vi "check operator action.vi"(9 "Motion Steps in":string[](array[string]), 10 "Part Type":string, 11 "input cluster":T3={"AT glass position"={"Tag Name"="S060.PXI.Signals.PlltData.SN", "Network Path"="172.15.51.1,1,0", "use opc"=FALSE, "DataSocket Reference"={"CWDSLib._DCWDataSocket"=refnum, "CWDSLib._DCWData"=refnum, "OnDataUpdated"=0, "OnStatusUpdated"=0}}, "AT shade position"={"Tag Name"="S060.PXI.Signals.PlltData.SN", "Network Path"="172.15.51.1,1,0", "use opc"=FALSE, "DataSocket Reference"={"CWDSLib._DCWDataSocket"=refnum, "CWDSLib._DCWData"=refnum, "OnDataUpdated"=0, "OnStatusUpdated"=0}}, "AT in glass wand lower pos"={"Tag Name"="S060.PXI.Signals.PlltData.SN", "Network Path"="172.15.51.1,1,0", "use opc"=FALSE, "DataSocket Reference"={"CWDSLib._DCWDataSocket"=refnum, "CWDSLib._DCWData"=refnum, "OnDataUpdated"=0, "OnStatusUpdated"=0}}, "AT in glass wand up pos"={"Tag Name"="S060.PXI.Signals.PlltData.SN", "Network Path"="172.15.51.1,1,0", "use opc"=FALSE, "DataSocket Reference"={"CWDSLib._DCWDataSocket"=refnum, "CWDSLib._DCWData"=refnum, "OnDataUpdated"=0, "OnStatusUpdated"=0}}, "AT in sunshad wand lower pos"={"Tag Name"="S060.PXI.Signals.PlltData.SN", "Network Path"="172.15.51.1,1,0", "use opc"=FALSE, "DataSocket Reference"={"CWDSLib._DCWDataSocket"=refnum, "CWDSLib._DCWData"=refnum, "OnDataUpdated"=0, "OnStatusUpdated"=0}}, "AT in sunshad wand up pos"={"Tag Name"="S060.PXI.Signals.PlltData.SN", "Network Path"="172.15.51.1,1,0", "use opc"=FALSE, "DataSocket Reference"={"CWDSLib._DCWDataSocket"=refnum, "CWDSLib._DCWData"=refnum, "OnDataUpdated"=0, "OnStatusUpdated"=0}}, "AT in wand home pos"={"Tag Name"="S060.PXI.Signals.PlltData.SN", "Network Path"="172.15.51.1,1,0", "use opc"=FALSE, "DataSocket Reference"={"CWDSLib._DCWDataSocket"=refnum, "CWDSLib._DCWData"=refnum, "OnDataUpdated"=0, "OnStatusUpdated"=0}}, "LVDT's Extended"={"Tag Name"="S060.PXI.Signals.PlltData.SN", "Network Path"="172.15.51.1,1,0", "use opc"=FALSE, "DataSocket Reference"={"CWDSLib._DCWDataSocket"=refnum, "CWDSLib._DCWData"=refnum, "OnDataUpdated"=0, "OnStatusUpdated"=0}}, "bolt check 1"={"Tag Name"="S060.PXI.Signals.PlltData.SN", "Network Path"="172.15.51.1,1,0", "use opc"=FALSE, "DataSocket Reference"={"CWDSLib._DCWDataSocket"=refnum, "CWDSLib._DCWData"=refnum, "OnDataUpdated"=0, "OnStatusUpdated"=0}}, "bolt check 2"={"Tag Name"="S060.PXI.Signals.PlltData.SN", "Network Path"="172.15.51.1,1,0", "use opc"=FALSE, "DataSocket Reference"={"CWDSLib._DCWDataSocket"=refnum, "CWDSLib._DCWData"=refnum, "OnDataUpdated"=0, "OnStatusUpdated"=0}}, "bolt check 3"={"Tag Name"="S060.PXI.Signals.PlltData.SN", "Network Path"="172.15.51.1,1,0", "use opc"=FALSE, "DataSocket Reference"={"CWDSLib._DCWDataSocket"=refnum, "CWDSLib._DCWData"=refnum, "OnDataUpdated"=0, "OnStatusUpdated"=0}}, "bolt check 4"={"Tag Name"="S060.PXI.Signals.PlltData.SN", "Network Path"="172.15.51.1,1,0", "use opc"=FALSE, "DataSocket Reference"={"CWDSLib._DCWDataSocket"=refnum, "CWDSLib._DCWData"=refnum, "OnDataUpdated"=0, "OnStatusUpdated"=0}}, "bolt check 5"={"Tag Name"="S060.PXI.Signals.PlltData.SN", "Network Path"="172.15.51.1,1,0", "use opc"=FALSE, "DataSocket Reference"={"CWDSLib._DCWDataSocket"=refnum, "CWDSLib._DCWData"=refnum, "OnDataUpdated"=0, "OnStatusUpdated"=0}}, "bolt check 6"={"Tag Name"="S060.PXI.Signals.PlltData.SN", "Network Path"="172.15.51.1,1,0", "use opc"=FALSE, "DataSocket Reference"={"CWDSLib._DCWDataSocket"=refnum, "CWDSLib._DCWData"=refnum, "OnDataUpdated"=0, "OnStatusUpdated"=0}}, "bolt check 7"={"Tag Name"="S060.PXI.Signals.PlltData.SN", "Network Path"="172.15.51.1,1,0", "use opc"=FALSE, "DataSocket Reference"={"CWDSLib._DCWDataSocket"=refnum, "CWDSLib._DCWData"=refnum, "OnDataUpdated"=0, "OnStatusUpdated"=0}}, "bolt check 8"={"Tag Name"="S060.PXI.Signals.PlltData.SN", "Network Path"="172.15.51.1,1,0", "use opc"=FALSE, "DataSocket Reference"={"CWDSLib._DCWDataSocket"=refnum, "CWDSLib._DCWData"=refnum, "OnDataUpdated"=0, "OnStatusUpdated"=0}}, "start"={"Tag Name"="S060.PXI.Signals.PlltData.SN", "Network Path"="172.15.51.1,1,0", "use opc"=FALSE, "DataSocket Reference"={"CWDSLib._DCWDataSocket"=refnum, "CWDSLib._DCWData"=refnum, "OnDataUpdated"=0, "OnStatusUpdated"=0}}, "abort"={"Tag Name"="S060.PXI.Signals.PlltData.SN", "Network Path"="172.15.51.1,1,0", "use opc"=FALSE, "DataSocket Reference"={"CWDSLib._DCWDataSocket"=refnum, "CWDSLib._DCWData"=refnum, "OnDataUpdated"=0, "OnStatusUpdated"=0}}, "LVDT's Retracted"={"Tag Name"="S060.PXI.Signals.PlltData.SN", "Network Path"="172.15.51.1,1,0", "use opc"=FALSE, "DataSocket Reference"={"CWDSLib._DCWDataSocket"=refnum, "CWDSLib._DCWData"=refnum, "OnDataUpdated"=0, "OnStatusUpdated"=0}}, "manual barcode print"={"Tag Name"="S060.PXI.Signals.PlltData.SN", "Network Path"="172.15.51.1,1,0", "use opc"=FALSE, "DataSocket Reference"={"CWDSLib._DCWDataSocket"=refnum, "CWDSLib._DCWData"=refnum, "OnDataUpdated"=0, "OnStatusUpdated"=0}}, "ss servo at open"={"Tag Name"="S060.PXI.Signals.PlltData.SN", "Network Path"="172.15.51.1,1,0", "use opc"=FALSE, "DataSocket Reference"={"CWDSLib._DCWDataSocket"=refnum, "CWDSLib._DCWData"=refnum, "OnDataUpdated"=0, "OnStatusUpdated"=0}}, "ss servo at close"={"Tag Name"="S060.PXI.Signals.PlltData.SN", "Network Path"="172.15.51.1,1,0", "use opc"=FALSE, "DataSocket Reference"={"CWDSLib._DCWDataSocket"=refnum, "CWDSLib._DCWData"=refnum, "OnDataUpdated"=0, "OnStatusUpdated"=0}}, "ss servo opening"={"Tag Name"="S060.PXI.Signals.PlltData.SN", "Network Path"="172.15.51.1,1,0", "use opc"=FALSE, "DataSocket Reference"={"CWDSLib._DCWDataSocket"=refnum, "CWDSLib._DCWData"=refnum, "OnDataUpdated"=0, "OnStatusUpdated"=0}}, "ss servo closing"={"Tag Name"="S060.PXI.Signals.PlltData.SN", "Network Path"="172.15.51.1,1,0", "use opc"=FALSE, "DataSocket Reference"={"CWDSLib._DCWDataSocket"=refnum, "CWDSLib._DCWData"=refnum, "OnDataUpdated"=0, "OnStatusUpdated"=0}}, "control slide at home"={"Tag Name"="S060.PXI.Signals.PlltData.SN", "Network Path"="172.15.51.1,1,0", "use opc"=FALSE, "DataSocket Reference"={"CWDSLib._DCWDataSocket"=refnum, "CWDSLib._DCWData"=refnum, "OnDataUpdated"=0, "OnStatusUpdated"=0}}, "control slide left good"={"Tag Name"="S060.PXI.Signals.PlltData.SN", "Network Path"="172.15.51.1,1,0", "use opc"=FALSE, "DataSocket Reference"={"CWDSLib._DCWDataSocket"=refnum, "CWDSLib._DCWData"=refnum, "OnDataUpdated"=0, "OnStatusUpdated"=0}}, "control slide left over stroke"={"Tag Name"="S060.PXI.Signals.PlltData.SN", "Network Path"="172.15.51.1,1,0", "use opc"=FALSE, "DataSocket Reference"={"CWDSLib._DCWDataSocket"=refnum, "CWDSLib._DCWData"=refnum, "OnDataUpdated"=0, "OnStatusUpdated"=0}}, "control slide right good"={"Tag Name"="S060.PXI.Signals.PlltData.SN", "Network Path"="172.15.51.1,1,0", "use opc"=FALSE, "DataSocket Reference"={"CWDSLib._DCWDataSocket"=refnum, "CWDSLib._DCWData"=refnum, "OnDataUpdated"=0, "OnStatusUpdated"=0}}, "control slide right over stroke"={"Tag Name"="S060.PXI.Signals.PlltData.SN", "Network Path"="172.15.51.1,1,0", "use opc"=FALSE, "DataSocket Reference"={"CWDSLib._DCWDataSocket"=refnum, "CWDSLib._DCWData"=refnum, "OnDataUpdated"=0, "OnStatusUpdated"=0}}, "wind deflector high speed pos"={"Tag Name"="S060.PXI.Signals.PlltData.SN", "Network Path"="172.15.51.1,1,0", "use opc"=FALSE, "DataSocket Reference"={"CWDSLib._DCWDataSocket"=refnum, "CWDSLib._DCWData"=refnum, "OnDataUpdated"=0, "OnStatusUpdated"=0}}, "wind deflector low speed pos"={"Tag Name"="S060.PXI.Signals.PlltData.SN", "Network Path"="172.15.51.1,1,0", "use opc"=FALSE, "DataSocket Reference"={"CWDSLib._DCWDataSocket"=refnum, "CWDSLib._DCWData"=refnum, "OnDataUpdated"=0, "OnStatusUpdated"=0}}, "AT VentPMACatHome"={"Tag Name"="S060.PXI.Signals.PlltData.SN", "Network Path"="172.15.51.1,1,0", "use opc"=FALSE, "DataSocket Reference"={"CWDSLib._DCWDataSocket"=refnum, "CWDSLib._DCWData"=refnum, "OnDataUpdated"=0, "OnStatusUpdated"=0}}, "AT VentPMACisExtend"={"Tag Name"="S060.PXI.Signals.PlltData.SN", "Network Path"="172.15.51.1,1,0", "use opc"=FALSE, "DataSocket Reference"={"CWDSLib._DCWDataSocket"=refnum, "CWDSLib._DCWData"=refnum, "OnDataUpdated"=0, "OnStatusUpdated"=0}}, "SS Barcode Scanner Bypassed"={"Tag Name"="S060.PXI.Signals.PlltData.SN", "Network Path"="172.15.51.1,1,0", "use opc"=FALSE, "DataSocket Reference"={"CWDSLib._DCWDataSocket"=refnum, "CWDSLib._DCWData"=refnum, "OnDataUpdated"=0, "OnStatusUpdated"=0}}, "Check Frame Barcode"={"Tag Name"="S060.PXI.Signals.PlltData.SN", "Network Path"="172.15.51.1,1,0", "use opc"=FALSE, "DataSocket Reference"={"CWDSLib._DCWDataSocket"=refnum, "CWDSLib._DCWData"=refnum, "OnDataUpdated"=0, "OnStatusUpdated"=0}}, "Z LVDTs Extended"={"Tag Name"="S060.PXI.Signals.PlltData.SN", "Network Path"="172.15.51.1,1,0", "use opc"=FALSE, "DataSocket Reference"={"CWDSLib._DCWDataSocket"=refnum, "CWDSLib._DCWData"=refnum, "OnDataUpdated"=0, "OnStatusUpdated"=0}}, "NVH Operator Pass"={"Tag Name"="S060.PXI.Signals.PlltData.SN", "Network Path"="172.15.51.1,1,0", "use opc"=FALSE, "DataSocket Reference"={"CWDSLib._DCWDataSocket"=refnum, "CWDSLib._DCWData"=refnum, "OnDataUpdated"=0, "OnStatusUpdated"=0}}, "NVH Operator Fail"={"Tag Name"="S060.PXI.Signals.PlltData.SN", "Network Path"="172.15.51.1,1,0", "use opc"=FALSE, "DataSocket Reference"={"CWDSLib._DCWDataSocket"=refnum, "CWDSLib._DCWData"=refnum, "OnDataUpdated"=0, "OnStatusUpdated"=0}}, "NVH Operator Express Glass Open"={"Tag Name"="S060.PXI.Signals.PlltData.SN", "Network Path"="172.15.51.1,1,0", "use opc"=FALSE, "DataSocket Reference"={"CWDSLib._DCWDataSocket"=refnum, "CWDSLib._DCWData"=refnum, "OnDataUpdated"=0, "OnStatusUpdated"=0}}, "NVH Operator Express Glass Close"={"Tag Name"="S060.PXI.Signals.PlltData.SN", "Network Path"="172.15.51.1,1,0", "use opc"=FALSE, "DataSocket Reference"={"CWDSLib._DCWDataSocket"=refnum, "CWDSLib._DCWData"=refnum, "OnDataUpdated"=0, "OnStatusUpdated"=0}}, "NVH Operator Express Rollo Open01"={"Tag Name"="S060.PXI.Signals.PlltData.SN", "Network Path"="172.15.51.1,1,0", "use opc"=FALSE, "DataSocket Reference"={"CWDSLib._DCWDataSocket"=refnum, "CWDSLib._DCWData"=refnum, "OnDataUpdated"=0, "OnStatusUpdated"=0}}, "NVH Operator Express Rollo Close01"={"Tag Name"="S060.PXI.Signals.PlltData.SN", "Network Path"="172.15.51.1,1,0", "use opc"=FALSE, "DataSocket Reference"={"CWDSLib._DCWDataSocket"=refnum, "CWDSLib._DCWData"=refnum, "OnDataUpdated"=0, "OnStatusUpdated"=0}}, "NVH Operator Express Rollo Open02"={"Tag Name"="S060.PXI.Signals.PlltData.SN", "Network Path"="172.15.51.1,1,0", "use opc"=FALSE, "DataSocket Reference"={"CWDSLib._DCWDataSocket"=refnum, "CWDSLib._DCWData"=refnum, "OnDataUpdated"=0, "OnStatusUpdated"=0}}, "NVH Operator Express Rollo Close02"={"Tag Name"="S060.PXI.Signals.PlltData.SN", "Network Path"="172.15.51.1,1,0", "use opc"=FALSE, "DataSocket Reference"={"CWDSLib._DCWDataSocket"=refnum, "CWDSLib._DCWData"=refnum, "OnDataUpdated"=0, "OnStatusUpdated"=0}}, "NVH Operator Vent Open Noise"={"Tag Name"="S060.PXI.Signals.PlltData.SN", "Network Path"="172.15.51.1,1,0", "use opc"=FALSE, "DataSocket Reference"={"CWDSLib._DCWDataSocket"=refnum, "CWDSLib._DCWData"=refnum, "OnDataUpdated"=0, "OnStatusUpdated"=0}}, "NVH Operator Vent Close Noise"={"Tag Name"="S060.PXI.Signals.PlltData.SN", "Network Path"="172.15.51.1,1,0", "use opc"=FALSE, "DataSocket Reference"={"CWDSLib._DCWDataSocket"=refnum, "CWDSLib._DCWData"=refnum, "OnDataUpdated"=0, "OnStatusUpdated"=0}}, "NVH Operator Sunshade Open Noise"={"Tag Name"="S060.PXI.Signals.PlltData.SN", "Network Path"="172.15.51.1,1,0", "use opc"=FALSE, "DataSocket Reference"={"CWDSLib._DCWDataSocket"=refnum, "CWDSLib._DCWData"=refnum, "OnDataUpdated"=0, "OnStatusUpdated"=0}}, "NVH Operator Sunshade Close Noise"={"Tag Name"="S060.PXI.Signals.PlltData.SN", "Network Path"="172.15.51.1,1,0", "use opc"=FALSE, "DataSocket Reference"={"CWDSLib._DCWDataSocket"=refnum, "CWDSLib._DCWData"=refnum, "OnDataUpdated"=0, "OnStatusUpdated"=0}}, "NVH Operator Glass Open Noise"={"Tag Name"="S060.PXI.Signals.PlltData.SN", "Network Path"="172.15.51.1,1,0", "use opc"=FALSE, "DataSocket Reference"={"CWDSLib._DCWDataSocket"=refnum, "CWDSLib._DCWData"=refnum, "OnDataUpdated"=0, "OnStatusUpdated"=0}}, "NVH Operator Glass Close Noise"={"Tag Name"="S060.PXI.Signals.PlltData.SN", "Network Path"="172.15.51.1,1,0", "use opc"=FALSE, "DataSocket Reference"={"CWDSLib._DCWDataSocket"=refnum, "CWDSLib._DCWData"=refnum, "OnDataUpdated"=0, "OnStatusUpdated"=0}}, "NVH Operator Finish"={"Tag Name"="S060.PXI.Signals.PlltData.SN", "Network Path"="172.15.51.1,1,0", "use opc"=FALSE, "DataSocket Reference"={"CWDSLib._DCWDataSocket"=refnum, "CWDSLib._DCWData"=refnum, "OnDataUpdated"=0, "OnStatusUpdated"=0}}, "NVH Operator Check"={"Tag Name"="S060.PXI.Signals.PlltData.SN", "Network Path"="172.15.51.1,1,0", "use opc"=FALSE, "DataSocket Reference"={"CWDSLib._DCWDataSocket"=refnum, "CWDSLib._DCWData"=refnum, "OnDataUpdated"=0, "OnStatusUpdated"=0}}, "windproof position"={"Tag Name"="S060.PXI.Signals.PlltData.SN", "Network Path"="172.15.51.1,1,0", "use opc"=FALSE, "DataSocket Reference"={"CWDSLib._DCWDataSocket"=refnum, "CWDSLib._DCWData"=refnum, "OnDataUpdated"=0, "OnStatusUpdated"=0}}, "NVH Operator Express Glass vent Open"={"Tag Name"="S060.PXI.Signals.PlltData.SN", "Network Path"="172.15.51.1,1,0", "use opc"=FALSE, "DataSocket Reference"={"CWDSLib._DCWDataSocket"=refnum, "CWDSLib._DCWData"=refnum, "OnDataUpdated"=0, "OnStatusUpdated"=0}}, "NVH Operator Express Glass Vent Close"={"Tag Name"="S060.PXI.Signals.PlltData.SN", "Network Path"="172.15.51.1,1,0", "use opc"=FALSE, "DataSocket Reference"={"CWDSLib._DCWDataSocket"=refnum, "CWDSLib._DCWData"=refnum, "OnDataUpdated"=0, "OnStatusUpdated"=0}}, "NVH Operator Re-do"={"Tag Name"="S060.PXI.Signals.PlltData.SN", "Network Path"="172.15.51.1,1,0", "use opc"=FALSE, "DataSocket Reference"={"CWDSLib._DCWDataSocket"=refnum, "CWDSLib._DCWData"=refnum, "OnDataUpdated"=0, "OnStatusUpdated"=0}}, "AT at vent ATS test pos"={"Tag Name"="S060.PXI.Signals.PlltData.SN", "Network Path"="172.15.51.1,1,0", "use opc"=FALSE, "DataSocket Reference"={"CWDSLib._DCWDataSocket"=refnum, "CWDSLib._DCWData"=refnum, "OnDataUpdated"=0, "OnStatusUpdated"=0}}, "AT at vent ATS Home pos"={"Tag Name"="S060.PXI.Signals.PlltData.SN", "Network Path"="172.15.51.1,1,0", "use opc"=FALSE, "DataSocket Reference"={"CWDSLib._DCWDataSocket"=refnum, "CWDSLib._DCWData"=refnum, "OnDataUpdated"=0, "OnStatusUpdated"=0}}, "Start Adjust LVDT"={"Tag Name"="S060.PXI.Signals.PlltData.SN", "Network Path"="172.15.51.1,1,0", "use opc"=FALSE, "DataSocket Reference"={"CWDSLib._DCWDataSocket"=refnum, "CWDSLib._DCWData"=refnum, "OnDataUpdated"=0, "OnStatusUpdated"=0}}, "Finish Adjust LVDT"={"Tag Name"="S060.PXI.Signals.PlltData.SN", "Network Path"="172.15.51.1,1,0", "use opc"=FALSE, "DataSocket Reference"={"CWDSLib._DCWDataSocket"=refnum, "CWDSLib._DCWData"=refnum, "OnDataUpdated"=0, "OnStatusUpdated"=0}}} {"AT in sunshad wand up pos"."DataSocket Reference"."OnStatusUpdated" format="%.0x"; "AT in sunshad wand up pos"."DataSocket Reference"."OnDataUpdated" format="%.0x"; "AT in glass wand up pos"."DataSocket Reference"."OnStatusUpdated" format="%.0x"; "AT in glass wand up pos"."DataSocket Reference"."OnDataUpdated" format="%.0x"; "Finish Adjust LVDT"."DataSocket Reference"."OnStatusUpdated" format="%.0x"; "Finish Adjust LVDT"."DataSocket Reference"."OnDataUpdated" format="%.0x"; "Start Adjust LVDT"."DataSocket Reference"."OnStatusUpdated" format="%.0x"; "Start Adjust LVDT"."DataSocket Reference"."OnDataUpdated" format="%.0x"; "AT at vent ATS Home pos"."DataSocket Reference"."OnStatusUpdated" format="%.0x"; "AT at vent ATS Home pos"."DataSocket Reference"."OnDataUpdated" format="%.0x"; "AT at vent ATS test pos"."DataSocket Reference"."OnStatusUpdated" format="%.0x"; "AT at vent ATS test pos"."DataSocket Reference"."OnDataUpdated" format="%.0x"; "NVH Operator Re-do"."DataSocket Reference"."OnStatusUpdated" format="%.0x"; "NVH Operator Re-do"."DataSocket Reference"."OnDataUpdated" format="%.0x"; "NVH Operator Express Glass Vent Close"."DataSocket Reference"."OnStatusUpdated" format="%.0x"; "NVH Operator Express Glass Vent Close"."DataSocket Reference"."OnDataUpdated" format="%.0x"; "NVH Operator Express Glass vent Open"."DataSocket Reference"."OnStatusUpdated" format="%.0x"; "NVH Operator Express Glass vent Open"."DataSocket Reference"."OnDataUpdated" format="%.0x"; "windproof position"."DataSocket Reference"."OnStatusUpdated" format="%.0x"; "windproof position"."DataSocket Reference"."OnDataUpdated" format="%.0x"; "NVH Operator Check"."DataSocket Reference"."OnStatusUpdated" format="%.0x"; "NVH Operator Check"."DataSocket Reference"."OnDataUpdated" format="%.0x"; "NVH Operator Finish"."DataSocket Reference"."OnStatusUpdated" format="%.0x"; "NVH Operator Finish"."DataSocket Reference"."OnDataUpdated" format="%.0x"; "NVH Operator Glass Close Noise"."DataSocket Reference"."OnStatusUpdated" format="%.0x"; "NVH Operator Glass Close Noise"."DataSocket Reference"."OnDataUpdated" format="%.0x"; "NVH Operator Glass Open Noise"."DataSocket Reference"."OnStatusUpdated" format="%.0x"; "NVH Operator Glass Open Noise"."DataSocket Reference"."OnDataUpdated" format="%.0x"; "NVH Operator Sunshade Close Noise"."DataSocket Reference"."OnStatusUpdated" format="%.0x"; "NVH Operator Sunshade Close Noise"."DataSocket Reference"."OnDataUpdated" format="%.0x"; "NVH Operator Sunshade Open Noise"."DataSocket Reference"."OnStatusUpdated" format="%.0x"; "NVH Operator Sunshade Open Noise"."DataSocket Reference"."OnDataUpdated" format="%.0x"; "NVH Operator Vent Close Noise"."DataSocket Reference"."OnStatusUpdated" format="%.0x"; "NVH Operator Vent Close Noise"."DataSocket Reference"."OnDataUpdated" format="%.0x"; "NVH Operator Vent Open Noise"."DataSocket Reference"."OnStatusUpdated" format="%.0x"; "NVH Operator Vent Open Noise"."DataSocket Reference"."OnDataUpdated" format="%.0x"; "NVH Operator Express Rollo Close02"."DataSocket Reference"."OnStatusUpdated" format="%.0x"; "NVH Operator Express Rollo Close02"."DataSocket Reference"."OnDataUpdated" format="%.0x"; "NVH Operator Express Rollo Open02"."DataSocket Reference"."OnStatusUpdated" format="%.0x"; "NVH Operator Express Rollo Open02"."DataSocket Reference"."OnDataUpdated" format="%.0x"; "NVH Operator Express Rollo Close01"."DataSocket Reference"."OnStatusUpdated" format="%.0x"; "NVH Operator Express Rollo Close01"."DataSocket Reference"."OnDataUpdated" format="%.0x"; "NVH Operator Express Rollo Open01"."DataSocket Reference"."OnStatusUpdated" format="%.0x"; "NVH Operator Express Rollo Open01"."DataSocket Reference"."OnDataUpdated" format="%.0x"; "NVH Operator Express Glass Close"."DataSocket Reference"."OnStatusUpdated" format="%.0x"; "NVH Operator Express Glass Close"."DataSocket Reference"."OnDataUpdated" format="%.0x"; "NVH Operator Express Glass Open"."DataSocket Reference"."OnStatusUpdated" format="%.0x"; "NVH Operator Express Glass Open"."DataSocket Reference"."OnDataUpdated" format="%.0x"; "NVH Operator Fail"."DataSocket Reference"."OnStatusUpdated" format="%.0x"; "NVH Operator Fail"."DataSocket Reference"."OnDataUpdated" format="%.0x"; "NVH Operator Pass"."DataSocket Reference"."OnStatusUpdated" format="%.0x"; "NVH Operator Pass"."DataSocket Reference"."OnDataUpdated" format="%.0x"; "Z LVDTs Extended"."DataSocket Reference"."OnStatusUpdated" format="%.0x"; "Z LVDTs Extended"."DataSocket Reference"."OnDataUpdated" format="%.0x"; "Check Frame Barcode"."DataSocket Reference"."OnStatusUpdated" format="%.0x"; "Check Frame Barcode"."DataSocket Reference"."OnDataUpdated" format="%.0x"; "SS Barcode Scanner Bypassed"."DataSocket Reference"."OnStatusUpdated" format="%.0x"; "SS Barcode Scanner Bypassed"."DataSocket Reference"."OnDataUpdated" format="%.0x"; "AT VentPMACisExtend"."DataSocket Reference"."OnStatusUpdated" format="%.0x"; "AT VentPMACisExtend"."DataSocket Reference"."OnDataUpdated" format="%.0x"; "AT VentPMACatHome"."DataSocket Reference"."OnStatusUpdated" format="%.0x"; "AT VentPMACatHome"."DataSocket Reference"."OnDataUpdated" format="%.0x"; "wind deflector low speed pos"."DataSocket Reference"."OnStatusUpdated" format="%.0x"; "wind deflector low speed pos"."DataSocket Reference"."OnDataUpdated" format="%.0x"; "wind deflector high speed pos"."DataSocket Reference"."OnStatusUpdated" format="%.0x"; "wind deflector high speed pos"."DataSocket Reference"."OnDataUpdated" format="%.0x"; "control slide right over stroke"."DataSocket Reference"."OnStatusUpdated" format="%.0x"; "control slide right over stroke"."DataSocket Reference"."OnDataUpdated" format="%.0x"; "control slide right good"."DataSocket Reference"."OnStatusUpdated" format="%.0x"; "control slide right good"."DataSocket Reference"."OnDataUpdated" format="%.0x"; "control slide left over stroke"."DataSocket Reference"."OnStatusUpdated" format="%.0x"; "control slide left over stroke"."DataSocket Reference"."OnDataUpdated" format="%.0x"; "control slide left good"."DataSocket Reference"."OnStatusUpdated" format="%.0x"; "control slide left good"."DataSocket Reference"."OnDataUpdated" format="%.0x"; "control slide at home"."DataSocket Reference"."OnStatusUpdated" format="%.0x"; "control slide at home"."DataSocket Reference"."OnDataUpdated" format="%.0x"; "ss servo closing"."DataSocket Reference"."OnStatusUpdated" format="%.0x"; "ss servo closing"."DataSocket Reference"."OnDataUpdated" format="%.0x"; "ss servo opening"."DataSocket Reference"."OnStatusUpdated" format="%.0x"; "ss servo opening"."DataSocket Reference"."OnDataUpdated" format="%.0x"; "ss servo at close"."DataSocket Reference"."OnStatusUpdated" format="%.0x"; "ss servo at close"."DataSocket Reference"."OnDataUpdated" format="%.0x"; "ss servo at open"."DataSocket Reference"."OnStatusUpdated" format="%.0x"; "ss servo at open"."DataSocket Reference"."OnDataUpdated" format="%.0x"; "manual barcode print"."DataSocket Reference"."OnStatusUpdated" format="%.0x"; "manual barcode print"."DataSocket Reference"."OnDataUpdated" format="%.0x"; "LVDT's Retracted"."DataSocket Reference"."OnStatusUpdated" format="%.0x"; "LVDT's Retracted"."DataSocket Reference"."OnDataUpdated" format="%.0x"; "abort"."DataSocket Reference"."OnStatusUpdated" format="%.0x"; "abort"."DataSocket Reference"."OnDataUpdated" format="%.0x"; "start"."DataSocket Reference"."OnStatusUpdated" format="%.0x"; "start"."DataSocket Reference"."OnDataUpdated" format="%.0x"; "bolt check 8"."DataSocket Reference"."OnStatusUpdated" format="%.0x"; "bolt check 8"."DataSocket Reference"."OnDataUpdated" format="%.0x"; "bolt check 7"."DataSocket Reference"."OnStatusUpdated" format="%.0x"; "bolt check 7"."DataSocket Reference"."OnDataUpdated" format="%.0x"; "bolt check 6"."DataSocket Reference"."OnStatusUpdated" format="%.0x"; "bolt check 6"."DataSocket Reference"."OnDataUpdated" format="%.0x"; "bolt check 5"."DataSocket Reference"."OnStatusUpdated" format="%.0x"; "bolt check 5"."DataSocket Reference"."OnDataUpdated" format="%.0x"; "bolt check 4"."DataSocket Reference"."OnStatusUpdated" format="%.0x"; "bolt check 4"."DataSocket Reference"."OnDataUpdated" format="%.0x"; "bolt check 3"."DataSocket Reference"."OnStatusUpdated" format="%.0x"; "bolt check 3"."DataSocket Reference"."OnDataUpdated" format="%.0x"; "bolt check 2"."DataSocket Reference"."OnStatusUpdated" format="%.0x"; "bolt check 2"."DataSocket Reference"."OnDataUpdated" format="%.0x"; "bolt check 1"."DataSocket Reference"."OnStatusUpdated" format="%.0x"; "bolt check 1"."DataSocket Reference"."OnDataUpdated" format="%.0x"; "LVDT's Extended"."DataSocket Reference"."OnStatusUpdated" format="%.0x"; "LVDT's Extended"."DataSocket Reference"."OnDataUpdated" format="%.0x"; "AT in wand home pos"."DataSocket Reference"."OnStatusUpdated" format="%.0x"; "AT in wand home pos"."DataSocket Reference"."OnDataUpdated" format="%.0x"; "AT in sunshad wand lower pos"."DataSocket Reference"."OnStatusUpdated" format="%.0x"; "AT in sunshad wand lower pos"."DataSocket Reference"."OnDataUpdated" format="%.0x"; "AT in glass wand lower pos"."DataSocket Reference"."OnStatusUpdated" format="%.0x"; "AT in glass wand lower pos"."DataSocket Reference"."OnDataUpdated" format="%.0x"; "AT shade position"."DataSocket Reference"."OnStatusUpdated" format="%.0x"; "AT shade position"."DataSocket Reference"."OnDataUpdated" format="%.0x"; "AT glass position"."DataSocket Reference"."OnStatusUpdated" format="%.0x"; "AT glass position"."DataSocket Reference"."OnDataUpdated" format="%.0x"}) -> (1 "Step":string, 2 "data string":string, 3 "Motion Steps out":string[](array[string]))   [LabVIEW 2018]
uses:
  02.Type Def's/station plc read boolean tags.ctl
  05.UserVI's/type defs/plc path and tag.ctl
  <vilib>/Platform/dataskt.llb/DataSocket Reference Type.ctl
  05.UserVI's/type defs/17x Audit Motion Data Seq Control.ctl
  05.UserVI's/type defs/17x AP Data Type.ctl
panel:
  in  "value":T1={"Power Supply Voltage"=13.5, "Min Avg Current"=0.0, "Max Avg Current"=0.0, "Min Run Time"=0.0, "Max Run Time"=0.0, "Min Speed"=0.0, "Max Speed"=0.0, "AP Data % of Threshold"=10.0, "Travel Distance"=0.0, "AP Data Type"=enum."91/61", "Check Current"=FALSE, "Check Run Time"=FALSE, "Check Speed"=FALSE, "Express Motion?"=FALSE, "Check Sound Test"=FALSE, "Check Position?"=FALSE, "Collect AP Data"=FALSE, "Inital Position"=0, "End Position"=0, "Goto Posiition"=0, "Max max Current"=0.0, "Min max Current"=0.0, "Check max Current"=FALSE, "Check Sound"=FALSE, "Min Sound (dB)"=0.0, "Max Sound (dB)"=0.0, "SW Mode"=enum."Hard Switch", "LIN Msg"={"ID"=0, "Msg"=[], "LDF"="EX1H"}} {"LIN Msg"."Msg" format="%02x"; "LIN Msg"."ID" format="%02x"}
  # "start/abort only used by barcode instance, since there are discrete signals for this in the other stations."
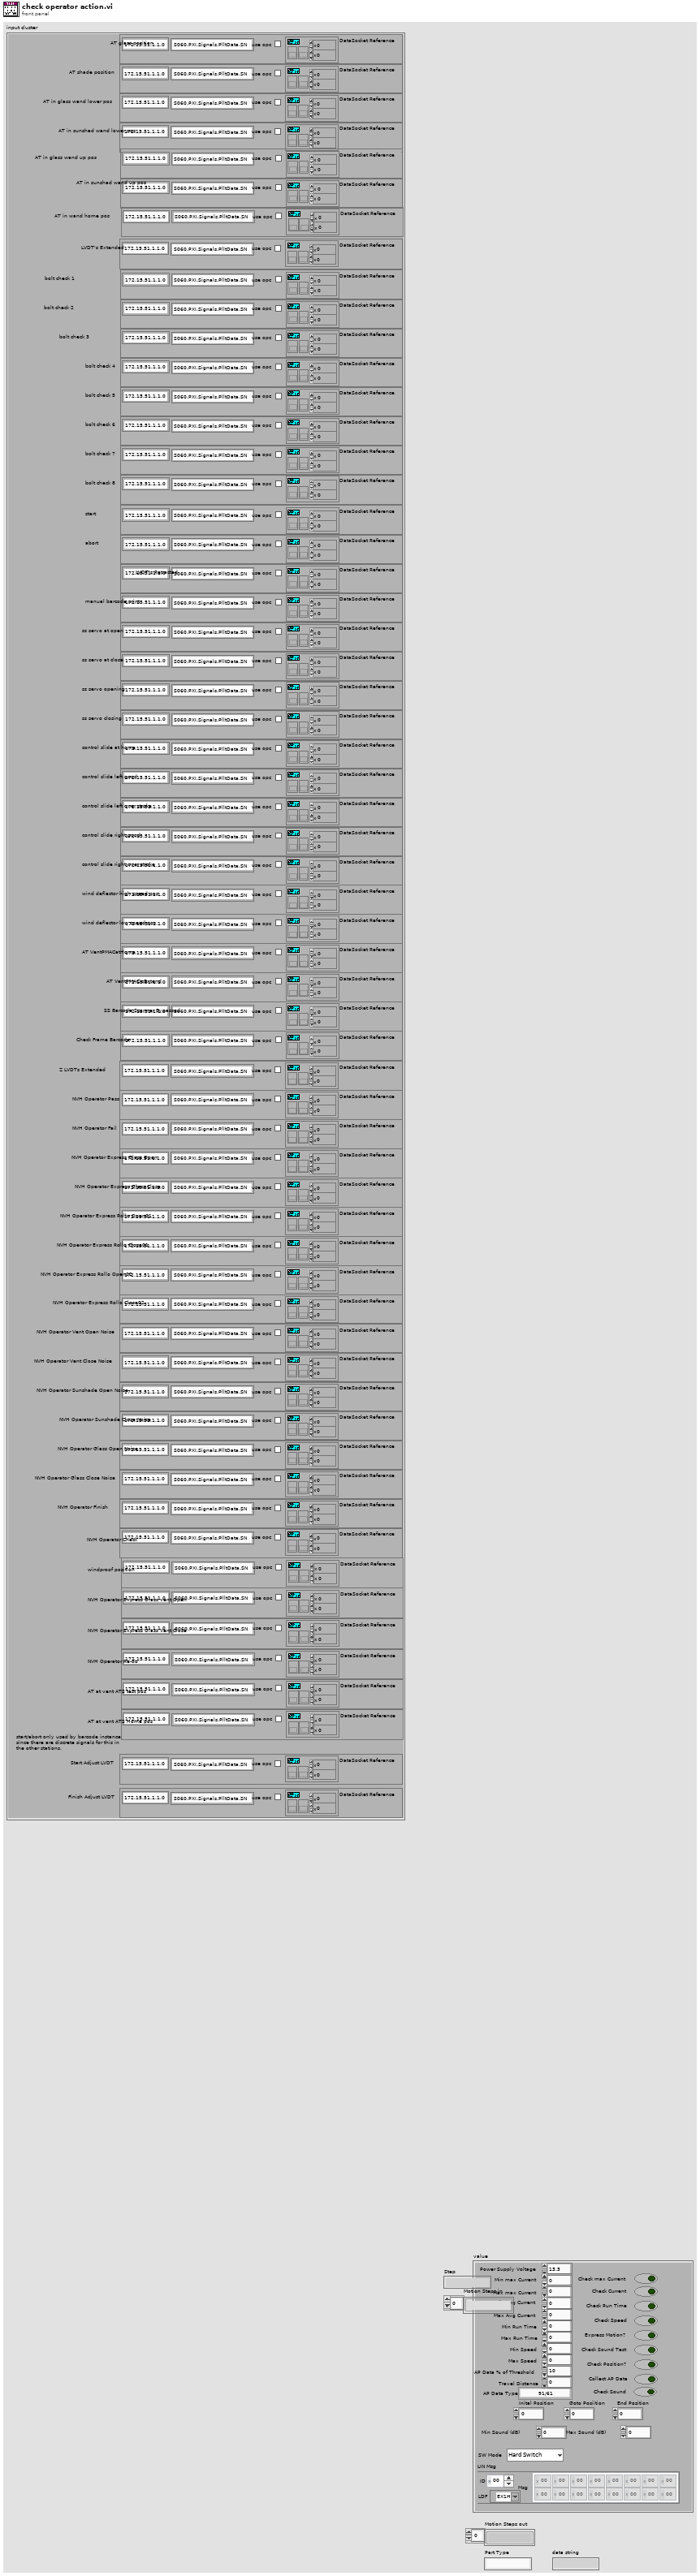
[diagram p1: front panel]
types:
  T1 = typedef "17x Audit Motion Data Seq Control.ctl" = cluster{"Power Supply Voltage":dbl, "Min Avg Current":dbl, "Max Avg Current":dbl, "Min Run Time":dbl, "Max Run Time":dbl, "Min Speed":dbl, "Max Speed":dbl, "AP Data % of Threshold":dbl, "Travel Distance":dbl, "AP Data Type":T2, "Check Current":bool, "Check Run Time":bool, "Check Speed":bool, "Express Motion?":bool, "Check Sound Test":bool, "Check Position?":bool, "Collect AP Data":bool, "Inital Position":u16, "End Position":u16, "Goto Posiition":u16, "Max max Current":dbl, "Min max Current":dbl, "Check max Current":bool, "Check Sound":bool, "Min Sound (dB)":dbl, "Max Sound (dB)":dbl, "SW Mode":enum16{"Hard Switch", "Uncond Frame"}, "LIN Msg":cluster{"ID":u8, "Msg":u8[][], "LDF":refnum<k21>}}
  T2 = typedef "17x AP Data Type.ctl" = enum16{"91/61", "92/62", "93/63", "67", "68", "6F", "71", "91 Msg", "92 Msg", "93 Msg", "94 Msg", "HiRain 91", "HiRain 92 Speed", "HiRain 92 HS", "HiRain 92", "HiRain 93", "SnT"}
  T3 = typedef "station plc read boolean tags.ctl" = cluster{"AT glass position":T4, "AT shade position":T4, "AT in glass wand lower pos":T4, "AT in glass wand up pos":T4, "AT in sunshad wand lower pos":T4, "AT in sunshad wand up pos":T4, "AT in wand home pos":T4, "LVDT's Extended":T4, "bolt check 1":T4, "bolt check 2":T4, "bolt check 3":T4, "bolt check 4":T4, "bolt check 5":T4, "bolt check 6":T4, "bolt check 7":T4, "bolt check 8":T4, "start":T4, "abort":T4, "LVDT's Retracted":T4, "manual barcode print":T4, "ss servo at open":T4, "ss servo at close":T4, "ss servo opening":T4, "ss servo closing":T4, "control slide at home":T4, "control slide left good":T4, "control slide left over stroke":T4, "control slide right good":T4, "control slide right over stroke":T4, "wind deflector high speed pos":T4, "wind deflector low speed pos":T4, "AT VentPMACatHome":T4, "AT VentPMACisExtend":T4, "SS Barcode Scanner Bypassed":T4, "Check Frame Barcode":T4, "Z LVDTs Extended":T4, "NVH Operator Pass":T4, "NVH Operator Fail":T4, "NVH Operator Express Glass Open":T4, "NVH Operator Express Glass Close":T4, "NVH Operator Express Rollo Open01":T4, "NVH Operator Express Rollo Close01":T4, "NVH Operator Express Rollo Open02":T4, "NVH Operator Express Rollo Close02":T4, "NVH Operator Vent Open Noise":T4, "NVH Operator Vent Close Noise":T4, "NVH Operator Sunshade Open Noise":T4, "NVH Operator Sunshade Close Noise":T4, "NVH Operator Glass Open Noise":T4, "NVH Operator Glass Close Noise":T4, "NVH Operator Finish":T4, "NVH Operator Check":T4, "windproof position":T4, "NVH Operator Express Glass vent Open":T4, "NVH Operator Express Glass Vent Close":T4, "NVH Operator Re-do":T4, "AT at vent ATS test pos":T4, "AT at vent ATS Home pos":T4, "Start Adjust LVDT":T4, "Finish Adjust LVDT":T4}
  T4 = typedef "plc path and tag.ctl" = cluster{"Tag Name":string, "Network Path":string, "use opc":bool, "DataSocket Reference":T5}
  T5 = typedef "DataSocket Reference Type.ctl" = cluster{"CWDSLib._DCWDataSocket":refnum<k7>, "CWDSLib._DCWData":refnum<k7>, "OnDataUpdated":u32, "OnStatusUpdated":u32}
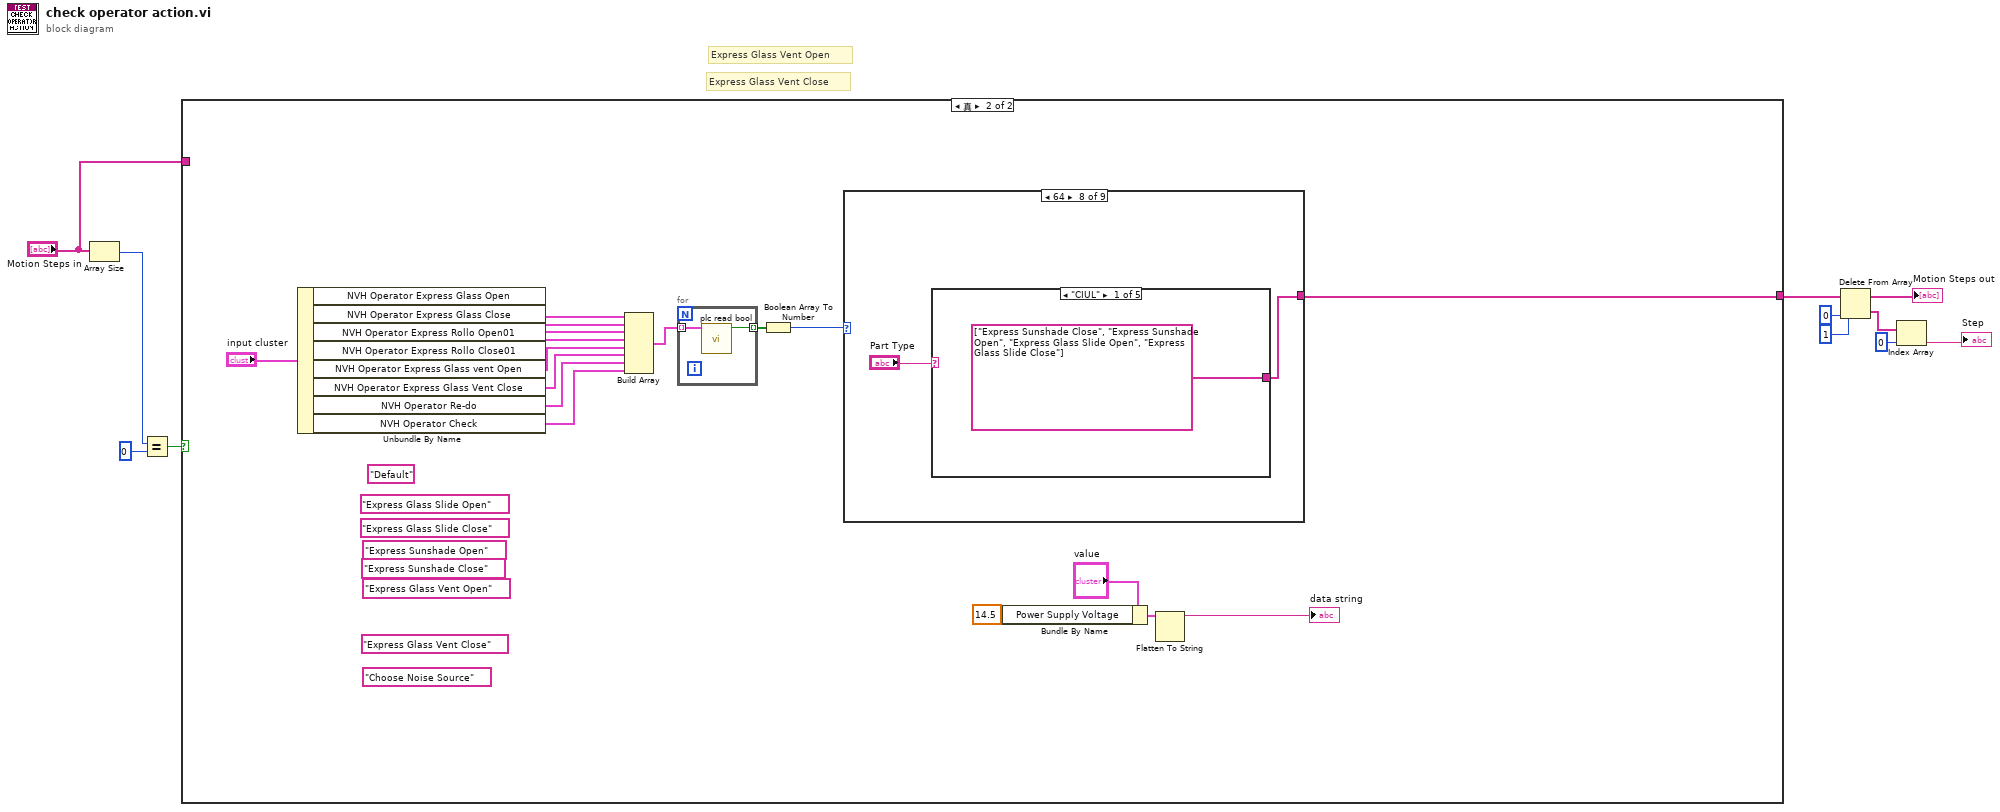
[diagram p0: block diagram]
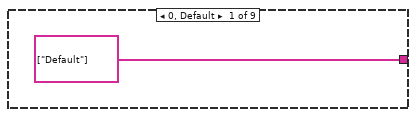
[diagram p3: hidden frame]
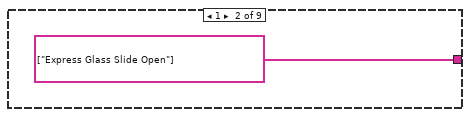
[diagram p4: hidden frame]
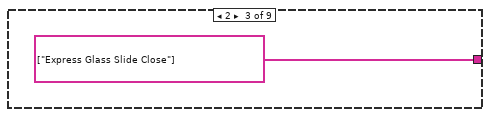
[diagram p5: hidden frame]
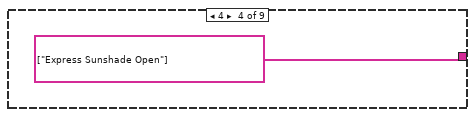
[diagram p6: hidden frame]
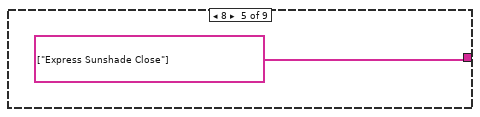
[diagram p7: hidden frame]
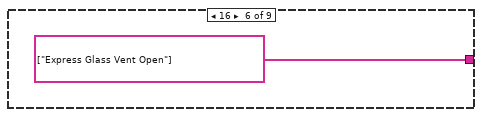
[diagram p8: hidden frame]
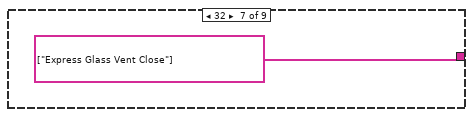
[diagram p9: hidden frame]
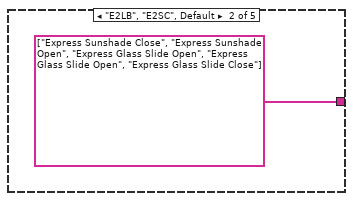
[diagram p10: hidden frame]
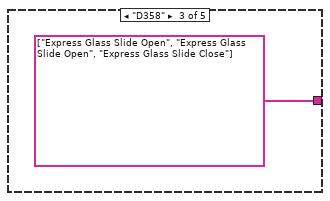
[diagram p11: hidden frame]
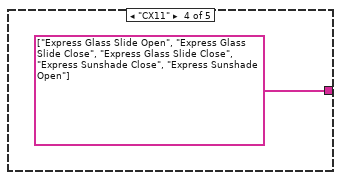
[diagram p12: hidden frame]
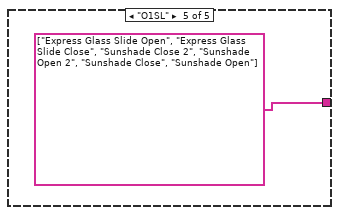
[diagram p13: hidden frame]
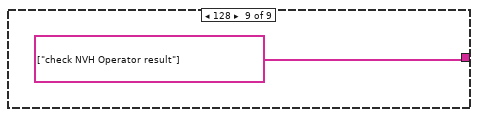
[diagram p14: hidden frame]
diagram:
  # "Express Glass Vent Open"
  # "Express Glass Vent Close"
  n1 = Array Size(array="Motion Steps in") -> (size(s)=w2:i32)
  n2 = Equal?(x=w2, y=0) -> (x = y?=w3:bool)
  n3 = case shown="真" w3 {
    tunnel: "Motion Steps in" -> [w12 _]
    tunnel: [w12 w13] -> w4
    frame False {
    }
    frame True {
      (unwired) "Choose Noise Source"
      (unwired) "Express Glass Vent Close"
      (unwired) "Express Glass Vent Open"
      (unwired) "Express Sunshade Close"
      (unwired) "Express Sunshade Open"
      (unwired) "Express Glass Slide Close"
      (unwired) "Express Glass Slide Open"
      (unwired) "Default"
      n4 = Unbundle By Name("input cluster") -> ("NVH Operator Express Glass Open"=w28:T4, "NVH Operator Express Glass Close"=w27:T4, "NVH Operator Express Rollo Open01"=w26:T4, "NVH Operator Express Rollo Close01"=w25:T4, "NVH Operator Express Glass vent Open"=w21:T4, "NVH Operator Express Glass Vent Close"=w16:T4, "NVH Operator Re-do"=w15:T4, "NVH Operator Check"=w14:T4)
      n5 = Build Array(w28, w27, w26, w25, w21, w16, w15, w14) -> (w24:T4[])
      n6 = for {
        tunnel: w24 -> [w46] mode=indexing
        tunnel: [w45] -> w23 mode=indexing
        n7 = call "plc read bool.vi"("addr,tag"=w46) -> ("value"=w45:bool)  [unwired: 9 in, 1 out]
      }
      n8 = Boolean Array To Number(Boolean array=w23) -> (number=w22:u32)
      n9 = case shown="64" w22 {
        tunnel: [string[] ["Default"] string[] ["Express Glass Slide Open"] string[] ["Express Glass Slide Close"] string[] ["Express Sunshade Open"] string[] ["Express Sunshade Close"] string[] ["Express Glass Vent Open"] string[] ["Express Glass Vent Close"] w37 string[] ["check NVH Operator result"]] -> w13
        frame 0, Default {
        }
        frame 1 {
        }
        frame 2 {
        }
        frame 4 {
        }
        frame 8 {
        }
        frame 16 {
        }
        frame 32 {
        }
        frame 64 {
          n10 = case shown="\"CIUL\"" "Part Type" {
            tunnel: [string[] ["Express Sunshade Close", "Express Sunshade Open", "Express Glass Slide Open", "Express Glass Slide Close"] string[] ["Express Sunshade Close", "Express Sunshade Open", "Express Glass Slide Open", "Express Glass Slide Open", "Express Glass Slide Close"] string[] ["Express Glass Slide Open", "Express Glass Slide Open", "Express Glass Slide Close"] string[] ["Express Glass Slide Open", "Express Glass Slide Close", "Express Glass Slide Close", "Express Sunshade Close", "Express Sunshade Open"] string[] ["Express Glass Slide Open", "Express Glass Slide Close", "Sunshade Close 2", "Sunshade Open 2", "Sunshade Close", "Sunshade Open"]] -> w37
            frame "CIUL" {
            }
            frame "E2LB", "E2SC", Default {
            }
            frame "D358" {
            }
            frame "CX11" {
            }
            frame "O1SL" {
            }
          }
        }
        frame 128 {
        }
      }
      n11 = Bundle By Name(cluster="value", "Power Supply Voltage"=14.5) -> (w17:T1)
      n12 = Flatten To String(anything=w17) -> (data string=→"data string":string)  [unwired: 3 in, 2 out]
    }
  }
  n13 = Delete From Array(array=w4, length=1, index=0) -> (deleted portion=w8:string[], array with subset deleted=→"Motion Steps out":string[])
  n14 = Index Array(array=w8, index=0) -> (element=→"Step":string)
